vi "Create Z Rotation Matrix.vi"(11 "Theta (°)":sgl) -> (3 "Rotation Z Matrix":sgl[][](array[numeric]))   [LabVIEW 2020, in "3D.lvlib"]
uses:
  3D.lvlib
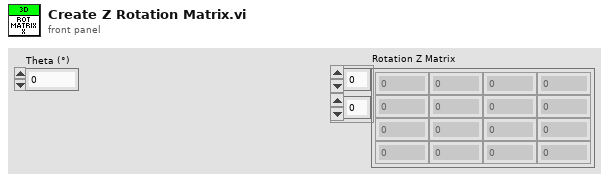
[diagram p1: front panel]
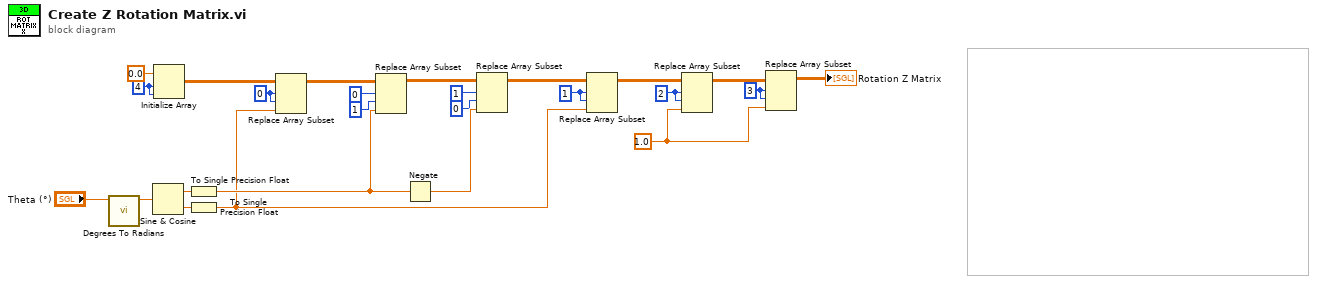
[diagram p0: block diagram]
diagram:
  w22 = sgl 1.0 ("new element/subarray")
  w21 = 3 ("index (row)")
  w19 = 2 ("index (row)")
  w18 = 1 ("index (row)")
  w9 = 0 ("index (row)")
  w8 = 4 ("dimension size")
  n1 = call "Degrees To Radians.vi"("Angle (°)"="Theta (°)") -> ("Angle (rad)"=w1:sgl)  [unwired: 10 in]
  n2 = Sine & Cosine(0:w1) -> (1:w6:sgl, 2:w4:sgl)
  n3 = Initialize Array(sgl 0.0 ("element"), w8, w8) -> (w25:sgl[][])
  n4 = To Single Precision Float(number=w6) -> (single precision float=w5:sgl)
  n5 = To Single Precision Float(number=w4) -> (single precision float=w3:sgl)
  n6 = Replace Array Subset(array=w25, new element=w3, index (row)=w9, index (col)=w9) -> (w10:sgl[][])
  n7 = Replace Array Subset(array=w10, new element=w5, index (row)=0, index (col)=1 ("disabled index (col)")) -> (w13:sgl[][])
  n8 = Negate(x=w5) -> (-x=w23:sgl)
  n9 = Replace Array Subset(array=w13, new element=w23, index (row)=1, index (col)=0 ("index (row)")) -> (w14:sgl[][])
  n10 = Replace Array Subset(array=w14, new element=w3, index (row)=w18, index (col)=w18) -> (w15:sgl[][])
  n11 = Replace Array Subset(array=w15, new element=w22, index (row)=w19, index (col)=w19) -> (w20:sgl[][])
  n12 = Replace Array Subset(array=w20, new element=w22, index (row)=w21, index (col)=w21) -> (→"Rotation Z Matrix":sgl[][])
